vi "Do Read.vi"(8 "error in (no error)":errorcluster, 10 "Interface":refnum<class "Interface.lvclass">, 11 "Section 2 in":refnum<class "Section 2.lvclass">) -> (0 "error out":errorcluster, 2 "All Keys Found?":bool, 3 "Section 2 out":refnum<class "Section 2.lvclass">)   [LabVIEW 2012, in "LVOOP Introduction.lvlib" / "Section 2.lvclass"]
doc: "Read keys/value pairs from Interface.\n\nOverwriting dynamic dispatch VI."
uses:
  Section 2.lvclass
  Configuration/Classes/Interface/Interface.lvclass
  Configuration/Classes/Section/Section.lvclass
  Section 2.lvclass/Section 2.ctl
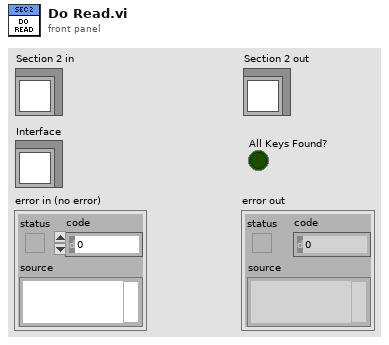
[diagram p1: front panel]
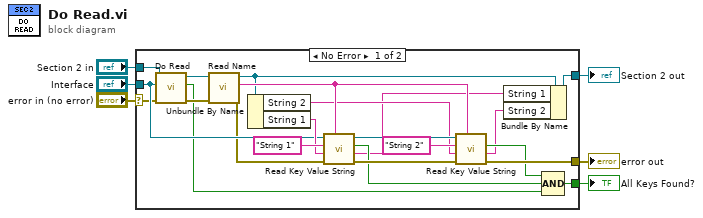
[diagram p0: block diagram]
diagram:
  n1 = case shown="No Error" "error in (no error)" {
    selector: "error in (no error)" -> [w8 w29]
    tunnel: "Section 2 in" -> [w28 w30]
    tunnel: [w20 w29] -> w5
    tunnel: [w18 w30] -> w4
    tunnel: "Interface" -> [w16 _]
    tunnel: [w11 _] -> w2
    frame No Error {
      n2 = call-parent "Do Read.vi"("error in (no error)"=w8, "Interface"=w16, "Section in"=w28) -> ("error out"=w17:errorcluster, "All Keys Found?"=w7:bool, "Section out"=w19:refnum<class "Section 2.lvclass">)  [unwired: 6 in]
      n3 = call "Read Name.vi"("error in (no error)"=w17, "Section in"=w19) -> ("error out"=w14:errorcluster, "Name"=w25:string, "Section out"=w22:refnum<class "Section 2.lvclass">)  [unwired: 7 in]
      n4 = Unbundle By Name(w22) -> ("String 2"=w15:string, "String 1"=w21:string)
      n5 = call-dynamic "Read Key Value String.vi"("Section Name"=w25, "error in (no error)"=w14, "Default"=w21, "Key Name"="String 1", "Interface in"=w16) -> ("error out"=w26:errorcluster, "Value"=w10:string, "found"=w12:bool, "Interface out"=w27:refnum<class "Interface.lvclass">)  [unwired: 3 in]
      n6 = call-dynamic "Read Key Value String.vi"("Section Name"=w25, "error in (no error)"=w26, "Default"=w15, "Key Name"="String 2", "Interface in"=w27) -> ("error out"=w20:errorcluster, "Value"=w9:string, "found"=w13:bool)  [unwired: 3 in, 1 out]
      n7 = Bundle By Name(cluster=w22, "String 1"=w10, "String 2"=w9) -> (w18:refnum<class "Section 2.lvclass">)
      n8 = Compound Arithmetic op=AND(w13, w12, w7) -> (w11:bool)
    }
    frame Error {
    }
  }
  "error out" <- w5
  "Section 2 out" <- w4
  "All Keys Found?" <- w2
